vi "Get File Name.vi"(8 "error in (no error)":errorcluster, 10 "Path":path, 11 "Function Generator Actor in":refnum<class "Function Generator Actor.lvclass">) -> (0 "error out":errorcluster, 3 "Function Generator Actor out":refnum<class "Function Generator Actor.lvclass">)   [LabVIEW 2020, in "Function Generator Actor.lvlib" / "Function Generator Actor.lvclass"]
uses:
  Function Generator Actor.lvclass
  Function Generator Actor.lvclass/Function Generator Actor.ctl
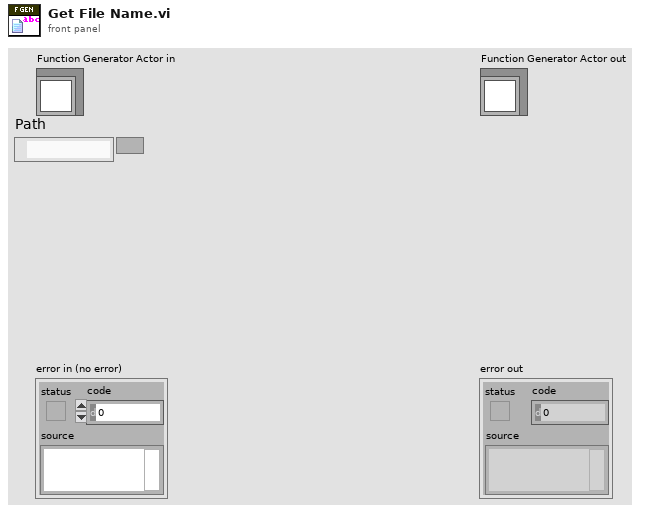
[diagram p1: front panel]
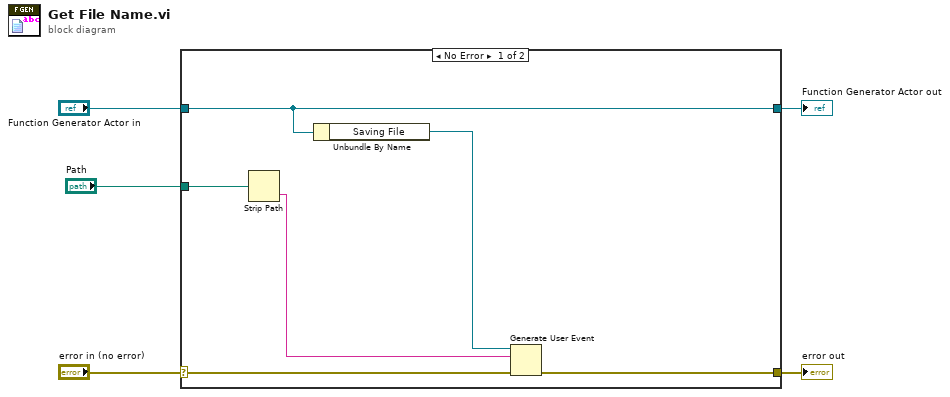
[diagram p0: block diagram]
diagram:
  n1 = case shown="No Error" "error in (no error)" {
    selector: "error in (no error)" -> [w10 w13]
    tunnel: [w9 w13] -> w4
    tunnel: [w8 w12] -> w2
    tunnel: "Function Generator Actor in" -> [w8 w12]
    tunnel: "Path" -> [w11 _]
    frame No Error {
      n2 = Strip Path(path=w11) -> (name=w6:string)  [unwired: 1 out]
      n3 = Unbundle By Name(w8) -> ("Saving File"=w7:refnum<user-event>)
      n4 = Generate User Event(user event=w7, event data cluster=w6, error in=w10) -> (error out=w9:errorcluster)  [unwired: 1 in, 1 out]
    }
    frame Error {
    }
  }
  "error out" <- w4
  "Function Generator Actor out" <- w2
